vi "ROS_Topic_Read_Primative.vi"(0 "ROS in":T1={"topic port"=0, "Node"="", "topic"="", "type"="", "node port"=0, "error "={"status"=FALSE, "code"=0, "source"=""}, "Direction"=enum."Node", "Update (ms)"=1, "FIFO size"=1}, 1 "Timeout (ms)":i32=500) -> (2 "ROS out":T1={"topic port"=0, "Node"="", "topic"="", "type"="", "node port"=0, "error "={"status"=FALSE, "code"=0, "source"=""}, "Direction"=enum."Node", "Update (ms)"=1, "FIFO size"=1}, 3 "timed out?":bool, 4 "Reply":string)   [LabVIEW 2016]
doc: "Returns any data received on the topic/service. Only use for subscribers or service clients. Data will need to be parsed."
uses:
  SubVIs/_ROSControl.ctl
  SubVIs/_ROSDirection.ctl
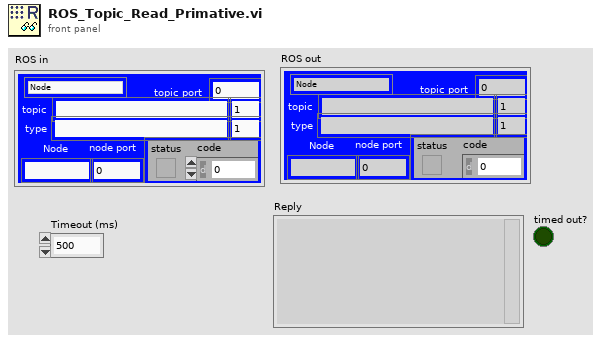
[diagram p1: front panel]
types:
  T1 = typedef "_ROSControl.ctl" = cluster{"topic port":u16, "Node":string, "topic":string, "type":string, "node port":u16, "error ":errorcluster, "Direction":T2, "Update (ms)":u16, "FIFO size":u16}
  T2 = typedef "_ROSDirection.ctl" = enum16{"Node", "Publisher", "Subscriber", "ServiceClient", "ServiceProvider"}
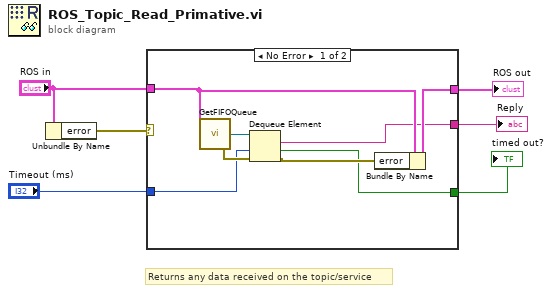
[diagram p0: block diagram]
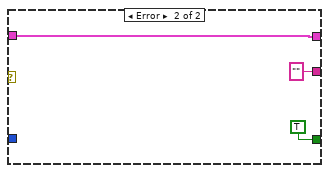
[diagram p2: hidden frame]
diagram:
  # "Returns any data received on the topic/service"
  n1 = Unbundle By Name("ROS in") -> ("error"=w2:errorcluster)
  n2 = case shown="No Error" w2 {
    tunnel: [w10 ""] -> w6
    tunnel: "Timeout (ms)" -> [w7 _]
    tunnel: [w14 w17] -> w4
    tunnel: "ROS in" -> [w13 w17]
    tunnel: [w9 TRUE ("timed out?")] -> w1
    frame No Error {
      n3 = call "GetFIFOQueue.vi"("ROS"=w13) -> ("error out"=w8:errorcluster, "queue out"=w12:refnum<queue>)  [unwired: 3 in]
      n4 = Dequeue Element(queue=w12, timeout in ms (-1)=w7, error in (no error)=w8) -> (element=w10:string, timed out?=w9:bool, error out=w11:errorcluster)  [unwired: 1 out]
      n5 = Bundle By Name(cluster=w13, "error"=w11) -> (w14:T1)
    }
    frame Error {
    }
  }
  "ROS out" <- w4
  "Reply" <- w6
  "timed out?" <- w1
